vi "Do.vi"(8 "error in (no error)":errorcluster, 10 "Actor in":refnum<class "Actor.lvclass">, 11 "Configure RTD [RTD] Msg":refnum<class "Configure RTD [RTD] Msg.lvclass">) -> (0 "error out":errorcluster, 2 "Actor out":refnum<class "Actor.lvclass">)   [LabVIEW 2015, in "CS++DMM.lvlib" / "Configure RTD [RTD] Msg.lvclass"]
doc: "This VI delivers the message to the actor by calling the appropriate method(s) on the actor."
uses:
  Configure RTD [RTD] Msg.lvclass
  CS++DMM/CS++DMM.lvclass
  CSPP_Core/Actors/CS++PVMonitor Messages/CS++PVUpdate Msg/CS++PVUpdate Msg.lvclass
  CSPP_Core/Classes/CS++ProcessVariables/ProcessVariable/PV.lvclass
  <vilib>/ActorFramework/Actor/Actor.lvclass
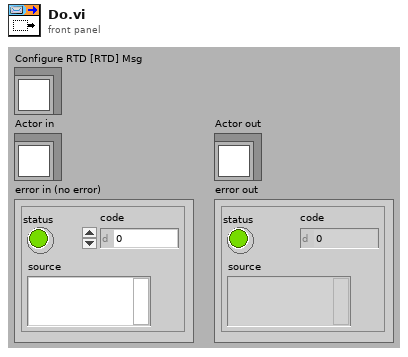
[diagram p1: front panel]
types:
  T1 = cluster{"alpha (0.0)":dbl, "resistance (0.0 ohms)":dbl}
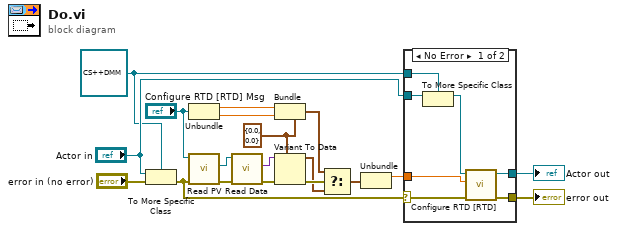
[diagram p0: block diagram]
diagram:
  w11 = T1 {"alpha (0.0)"=0.0, "resistance (0.0 ohms)"=0.0} ("Type")
  w15 = refnum<class "CS++DMM.lvclass"> refnum ("Actor in")
  n1 = To More Specific Class(target class=w15, reference="Actor in", error in="error in (no error)") -> (error out=w4:errorcluster)  [unwired: 1 out]
  n2 = Unbundle ("Pre-Unbundler")("Configure RTD [RTD] Msg") -> (w2:dbl, w1:dbl)
  n3 = call "Read PV.vi"("error in (no error)"=w4, "CS++PVUpdate Msg in"="Configure RTD [RTD] Msg") -> ("error out"=w14:errorcluster, "PV"=w10:refnum<class "PV.lvclass">)  [unwired: 7 in, 1 out]
  n4 = call "Read Data.vi"("error in (no error)"=w14, "PV in"=w10) -> ("error out"=w8:errorcluster, "Data"=w9:variant)  [unwired: 7 in, 1 out]
  n5 = Bundle ("Pre-Bundler")(cluster=w11, "alpha (0.0)"=w2, "resistance (0.0 ohms)"=w1) -> (w12:T1)
  n6 = Variant To Data(error in=w8, type=w11, Variant=w9) -> (data=w6:T1, error out=w13:errorcluster)
  n7 = Select ("MainSelect")(t=w12, s=w13, f=w6) -> (s? t:f=w7:T1)
  n8 = Unbundle ("Main-Unbundler")(w7) -> ("alpha (0.0)"=w3:dbl)  [unwired: 1 out]
  n9 = case shown="No Error" w4 {
    selector: w4 -> [w24 w28]
    tunnel: [w26 w28] -> w18
    tunnel: [w25 w27] -> w17
    tunnel: "Actor in" -> [w23 w27]
    tunnel: w15 -> [w22 _]
    tunnel: w3 -> [w20 _]
    frame No Error {
      n10 = To More Specific Class(target class=w22, reference=w23) -> (specific class reference=w21:refnum<class "CS++DMM.lvclass">)  [unwired: 1 in, 1 out]
      n11 = call "Configure RTD [RTD].vi"("error in (no error)"=w24, "alpha (0.0)"=w20, "CS++DMM in"=w21) -> ("error out"=w26:errorcluster, "CS++DMM out"=w25:refnum<class "CS++DMM.lvclass">)  [unwired: 7 in]
    }
    frame Error {
    }
  }
  "error out" <- w18
  "Actor out" <- w17
